vi "analysis_TimeResponse.vi"(11 "Time Response Parametric Data":T1) -> (1 "ST":dbl[](array[numeric]), 2 "PT":dbl[](array[numeric]), 3 "RT":dbl[](array[numeric]), 4 "OS":dbl[](array[numeric]), 5 "PV":dbl[](array[numeric]), 6 "SSG":dbl[](array[numeric]))   [LabVIEW 2017]
uses:
  <vilib>/addons/Control Design/_Model Construction/Data Typedefs.llb/CD Parametric Time Response Data.ctl
  <vilib>/addons/Control Design/_Model Construction/NI_LinSys_Data Typedefs.lvlib
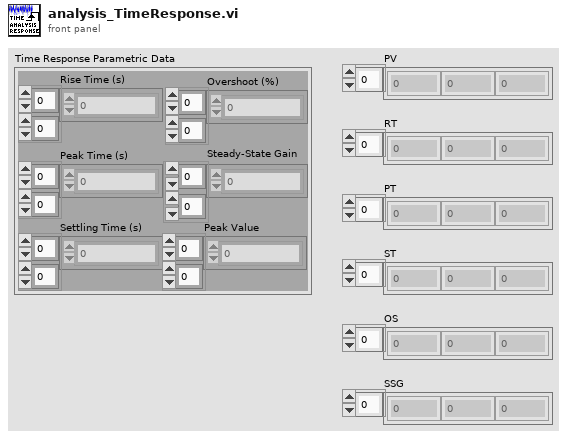
[diagram p1: front panel]
types:
  T1 = typedef "NI_LinSys_Data Typedefs.lvlib/CD Parametric Time Response Data.ctl" = cluster{"Rise Time (s)":dbl[][], "Peak Time (s)":dbl[][], "Settling Time (s)":dbl[][], "Overshoot (%)":dbl[][], "Steady-State Gain":dbl[][], "Peak Value":dbl[][]}
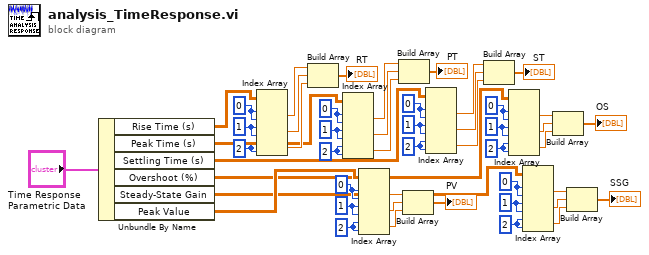
[diagram p0: block diagram]
diagram:
  w46 = 2 ("index (row)")
  w47 = 1 ("index (row)")
  w49 = 0 ("index (row)")
  w35 = 2 ("index (row)")
  w34 = 1 ("index (row)")
  w36 = 0 ("index (row)")
  w31 = 2 ("index (row)")
  w33 = 1 ("index (row)")
  w30 = 0 ("index (row)")
  w10 = 2 ("index (row)")
  w11 = 1 ("index (row)")
  w12 = 0 ("index (row)")
  w8 = 2 ("index (row)")
  w7 = 1 ("index (row)")
  w6 = 0 ("index (row)")
  w5 = 2 ("index (row)")
  w4 = 1 ("index (row)")
  w3 = 0 ("index (row)")
  n1 = Unbundle By Name("Time Response Parametric Data") -> ("Rise Time (s)"=w1:dbl[][], "Peak Time (s)"=w9:dbl[][], "Settling Time (s)"=w13:dbl[][], "Overshoot (%)"=w32:dbl[][], "Steady-State Gain"=w41:dbl[][], "Peak Value"=w48:dbl[][])
  n2 = Index Array(array=w1, index (row) #1=w3, index (col) #1=w3, index (row) #2=w4, index (col) #2=w4, index (row) #3=w5, index (col) #3=w5) -> (element #1=w16:dbl, element #2=w17:dbl, element #3=w18:dbl)
  n3 = Build Array(w16, w17, w18) -> (→"RT":dbl[])
  n4 = Index Array(array=w9, index (row) #1=w6, index (col) #1=w6, index (row) #2=w7, index (col) #2=w7, index (row) #3=w8, index (col) #3=w8) -> (element #1=w21:dbl, element #2=w22:dbl, element #3=w23:dbl)
  n5 = Index Array(array=w48, index (row) #1=w49, index (col) #1=w49, index (row) #2=w47, index (col) #2=w47, index (row) #3=w46, index (col) #3=w46) -> (element #1=w45:dbl, element #2=w44:dbl, element #3=w43:dbl)
  n6 = Build Array(w21, w22, w23) -> (→"PT":dbl[])
  n7 = Build Array(w45, w44, w43) -> (→"PV":dbl[])
  n8 = Index Array(array=w13, index (row) #1=w12, index (col) #1=w12, index (row) #2=w11, index (col) #2=w11, index (row) #3=w10, index (col) #3=w10) -> (element #1=w14:dbl, element #2=w15:dbl, element #3=w19:dbl)
  n9 = Build Array(w14, w15, w19) -> (→"ST":dbl[])
  n10 = Index Array(array=w32, index (row) #1=w30, index (col) #1=w30, index (row) #2=w33, index (col) #2=w33, index (row) #3=w31, index (col) #3=w31) -> (element #1=w29:dbl, element #2=w28:dbl, element #3=w27:dbl)
  n11 = Index Array(array=w41, index (row) #1=w36, index (col) #1=w36, index (row) #2=w34, index (col) #2=w34, index (row) #3=w35, index (col) #3=w35) -> (element #1=w37:dbl, element #2=w38:dbl, element #3=w39:dbl)
  n12 = Build Array(w29, w28, w27) -> (→"OS":dbl[])
  n13 = Build Array(w37, w38, w39) -> (→"SSG":dbl[])
